vi "Read Disconnected.vi"(8 "error in (no error)":errorcluster, 11 "WAMP Client in":refnum<class "WAMP Client.lvclass">) -> (0 "error out":errorcluster, 2 "Disconnected":refnum<user-event>, 3 "WAMP Client out":refnum<class "WAMP Client.lvclass">)   [LabVIEW 2020, in "wamplv.lvlib" / "WAMP Client.lvclass"]
uses:
  WAMP Client.lvclass
  WAMP Client.lvclass/WAMP Client.ctl
  Private/Events/EventsParent/Events.lvclass
  Private/TypeDef/Termination Reason Enum.ctl
  API/TypeDefs/Termination Reason.ctl
  wamplv.lvlib
  API/TypeDefs/Disconnected event data.ctl
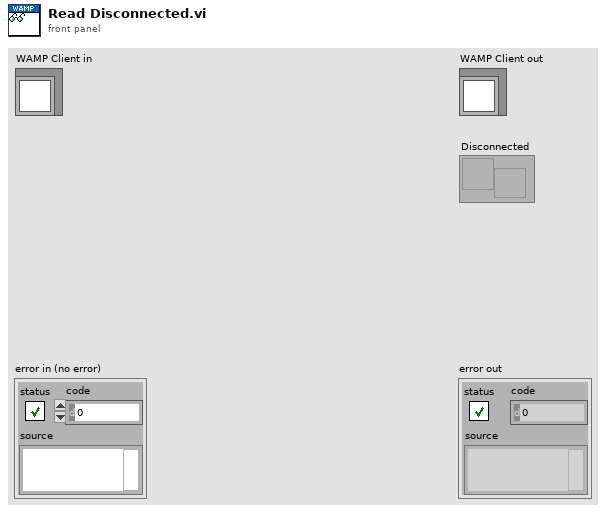
[diagram p1: front panel]
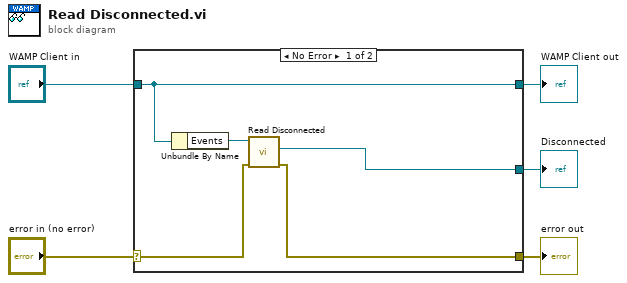
[diagram p0: block diagram]
diagram:
  n1 = case shown="No Error" "error in (no error)" {
    selector: "error in (no error)" -> [w7 w11]
    tunnel: [w6 w11] -> w4
    tunnel: [w10 w12] -> w2
    tunnel: "WAMP Client in" -> [w10 w12]
    tunnel: [w8 _] -> w1
    frame No Error {
      n2 = Unbundle By Name(w10) -> ("Events"=w9:refnum<class "Events.lvclass">)
      n3 = call "Read Disconnected.vi"("error in (no error)"=w7, "EventsParent in"=w9) -> ("error out"=w6:errorcluster, "Disconnected"=w8:refnum<user-event>)  [unwired: 7 in, 1 out]
    }
    frame Error {
    }
  }
  "error out" <- w4
  "WAMP Client out" <- w2
  "Disconnected" <- w1
